vi "Begin.vi"() -> (0 "error out":errorcluster)   [LabVIEW 2013]
doc: "Called before other user functions, this VI is expected to open initial I/O refnums, load in file data, and do all program initialization. Notice that the <B>error out</B> terminal is simply used for data flow. Wiring it to other structures or subVIs ensures that this VI runs first."
uses:
  <vilib>/Rock Robotics/WPI/Camera/WPI_CameraWhite Balance Values.ctl
  <vilib>/Rock Robotics/WPI/Camera/WPI_CameraExposure Values.ctl
  <vilib>/Rock Robotics/WPI/Camera/WPI_CameraFrameRate.ctl
  <vilib>/Rock Robotics/WPI/Camera/WPI_CameraImageSize.ctl
  Robot Global Data.vi
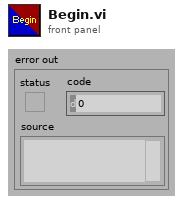
[diagram p1: front panel]
types:
  T1 = typedef "WPI_CameraImageSize.ctl" = enum16{"640x480", "320x240", "160x120"}
  T2 = typedef "WPI_CameraFrameRate.ctl" = u32
  T3 = typedef "WPI_CameraExposure Values.ctl" = enum16{"Auto", "Flicker-free 50 Hz", "Flicker-free 60 Hz", "Hold current"}
  T4 = typedef "WPI_CameraWhite Balance Values.ctl" = enum16{"Auto", "Fixed indoor", "Fixed outdoor 1", "Fixed outdoor 2", "Fixed fluorescent 1", "Fixed fluorescent 2", "Hold current"}
  T5 = typedef "WPI_CameraDevRef.ctl" = cluster{"Camera Address":string, "CameraStatus":errorcluster, "Acquire Image Notifier":refnum<notifier>}
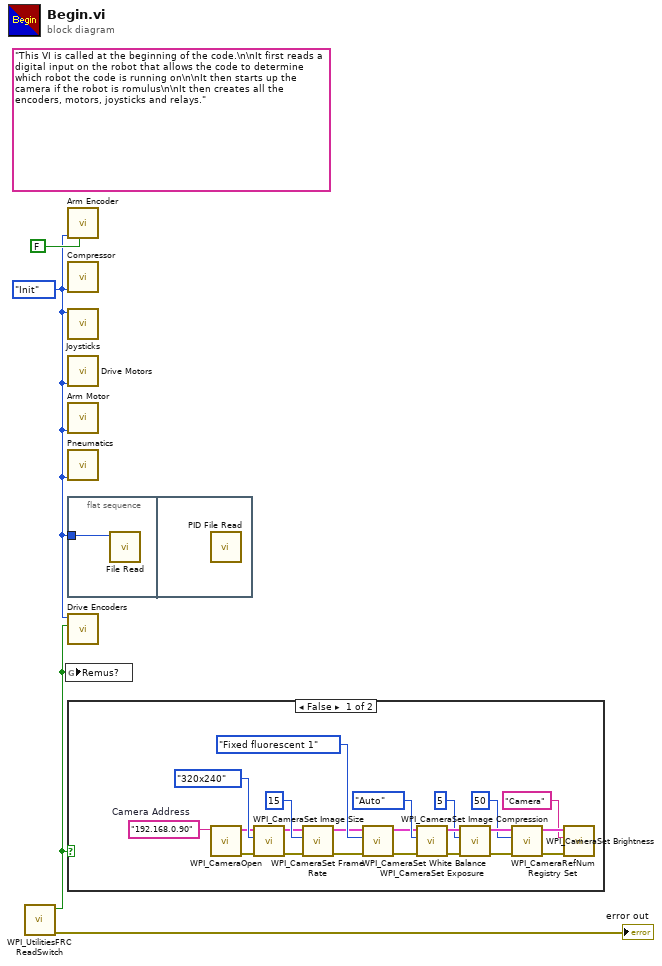
[diagram p0: block diagram]
diagram:
  w1 = enum16{"Init", "Run", "End"}."Init" ("Mode")
  (unwired) "This VI is called at the beginning of the code.\n\nIt first reads a digital input on the robot that allows the code to determine which robot the code is running on\n\nIt then starts up the camera if the robot is romulus\n\nIt then creates all the encoders, motors, joysticks and relays."
  n1 = call <vilib>:"WPI_UtilitiesFRC ReadSwitch.vi"() -> ("error out"=→"error out":errorcluster, "switch state"=w3:bool)  [unwired: 1 in, 9 out]
  n2 = global write "Robot Global Data.vi" "Remus?"(w3) -> ()
  n3 = call "Arm Encoder.vi"("Reset Encoder?"=FALSE, "Mode"=w1) -> ()  [unwired: 1 in, 9 out]
  n4 = call "Compressor.vi"("Mode"=w1) -> ()  [unwired: 3 in, 8 out]
  n5 = call "Joysticks.vi"("Mode"=w1) -> ()  [unwired: 9 out]
  n6 = call "Drive Motors.vi"("Mode"=w1) -> ()  [unwired: 2 in, 9 out]
  n7 = call "Arm Motor.vi"("Mode"=w1) -> ()  [unwired: 3 in, 8 out]
  n8 = call "Pneumatics.vi"("Mode"=w1) -> ()  [unwired: 2 in, 9 out]
  n9 = flat-sequence {
    tunnel: w1 -> [w5]
    frame #0 {
      n10 = call "File Read.vi"("Mode"=w5) -> ()  [unwired: 2 in, 9 out]
    }
    frame #1 {
      n11 = call "PID File Read.vi"() -> ()  [unwired: 1 out]
    }
  }
  n12 = call "Drive Encoders.vi"("Remus?"=w3, "Mode"=w1) -> ()  [unwired: 2 in, 8 out]
  n13 = case shown="False" w3 {
    frame False {
      w6 = "192.168.0.90"  # Camera Address
      n14 = call <vilib>:"WPI_CameraOpen.vi"("Camera Address"=w6) -> ("error out"=w16:errorcluster, "CameraDevRef"=w15:T5)  [unwired: 1 in, 8 out]
      n15 = call <vilib>:"WPI_CameraSet Image Size.vi"("error in (no error)"=w16, "Image Size"=WPI_CameraImageSize."320x240", "CameraDevRef"=w15) -> ("error out"=w17:errorcluster, "CameraDevRef Out"=w14:T5)  [unwired: 7 out]
      n16 = call <vilib>:"WPI_CameraSet Frame Rate.vi"("error in (no error)"=w17, "Frame Rate (fps)"=T2 15, "CameraDevRef"=w14) -> ("error out"=w18:errorcluster, "CameraDevRef Out"=w12:T5)  [unwired: 7 out]
      n17 = call <vilib>:"WPI_CameraSet White Balance.vi"("error in (no error)"=w18, "White Balance"=WPI_CameraWhite_Balance_Values."Fixed fluorescent 1", "CameraDevRef"=w12) -> ("error out"=w19:errorcluster, "CameraDevRef Out"=w13:T5)  [unwired: 7 out]
      n18 = call <vilib>:"WPI_CameraSet Exposure.vi"("error in (no error)"=w19, "Exposure"=WPI_CameraExposure_Values."Auto", "CameraDevRef"=w13) -> ("error out"=w20:errorcluster, "CameraDevRef Out"=w10:T5)  [unwired: 7 out]
      n19 = call <vilib>:"WPI_CameraSet Image Compression.vi"("error in (no error)"=w20, "Compression"=5, "CameraDevRef"=w10) -> ("error out"=w21:errorcluster, "CameraDevRef Out"=w11:T5)  [unwired: 7 out]
      n20 = call <vilib>:"WPI_CameraSet Brightness.vi"("error in (no error)"=w21, "Brightness"=50, "CameraDevRef"=w11) -> ("error out"=w23:errorcluster, "CameraDevRef Out"=w22:T5)  [unwired: 7 out]
      n21 = call <vilib>:"WPI_CameraRefNum Registry Set.vi"("error in (no error)"=w23, "refnum name"="Camera", "CameraDevRef"=w22) -> ()  [unwired: 9 out]
    }
    frame True {
    }
  }
